vi "interlock_TEST_LOGIC.vi"(4 "DRIVER_PCB":string, 5 "LB_PCB":string, 6 "FPL_PCB":string, 7 "HB_PCB":string, 8 "DRIVER_PCB":string[](array[string]), 9 "FPL_PCB":string[](array[string]), 10 "LB_PCB":string[](array[string]), 11 "HB_PCB":string[](array[string])) -> (0 "DRIVER_PCB":bool, 1 "FPL_PCB":bool, 2 "LB_PCB":bool, 3 "HB_PCB":bool)   [LabVIEW 2017]
panel:
  in  "table":string[][](table)=[["ss", "ss", "ss", "ss"], ["ddd", "ddd", "dasss", "sssssww"], ["sumit", "Amit", "Atual", "Shital"], ["S", "S", "S", "S"]]
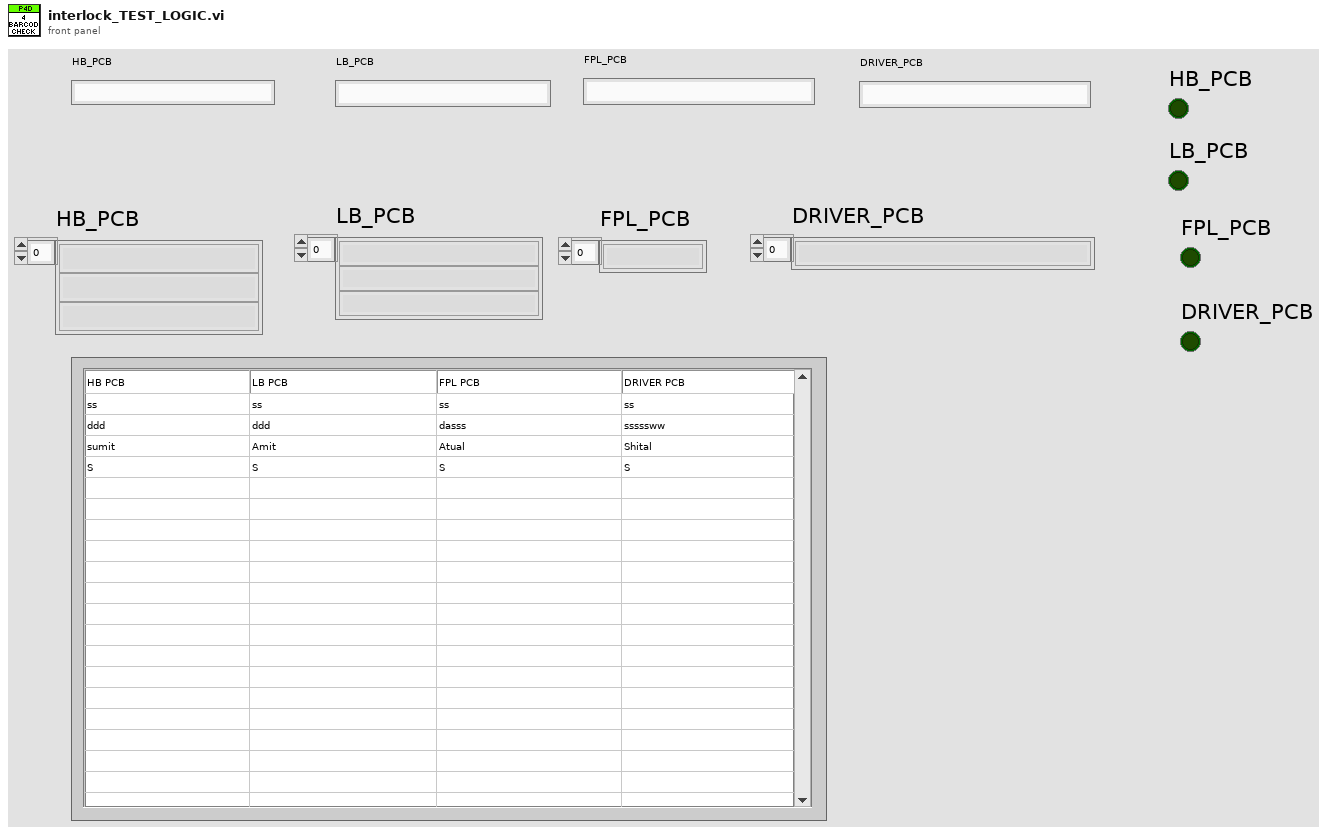
[diagram p1: front panel]
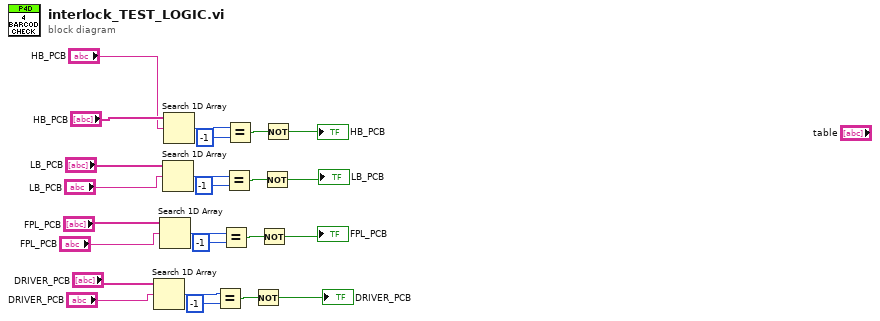
[diagram p0: block diagram]
diagram:
  n1 = Search 1D Array(1D array="DRIVER_PCB", element="DRIVER_PCB") -> (index of element=w2:i32)  [unwired: 1 in]
  n2 = Search 1D Array(1D array="FPL_PCB", element="FPL_PCB") -> (index of element=w1:i32)  [unwired: 1 in]
  n3 = Search 1D Array(1D array="LB_PCB", element="LB_PCB") -> (index of element=w17:i32)  [unwired: 1 in]
  n4 = Search 1D Array(1D array="HB_PCB", element="HB_PCB") -> (index of element=w24:i32)  [unwired: 1 in]
  n5 = Equal?(x=w2, y=-1) -> (x = y?=w14:bool)
  n6 = Equal?(x=w1, y=-1) -> (x = y?=w15:bool)
  n7 = Equal?(x=w17, y=-1) -> (x = y?=w19:bool)
  n8 = Equal?(x=w24, y=-1) -> (x = y?=w22:bool)
  n9 = Not(x=w14) -> (.not. x?=→"DRIVER_PCB":bool)
  n10 = Not(x=w15) -> (.not. x?=→"FPL_PCB":bool)
  n11 = Not(x=w19) -> (.not. x?=→"LB_PCB":bool)
  n12 = Not(x=w22) -> (.not. x?=→"HB_PCB":bool)
